vi "angle_sensor.vi"() -> (0 "Angle of system":dbl)   [LabVIEW 2014]
uses:
  <vilib>/myRIO/Instrument Drivers/Onboard IO/AI/typedefs/AI Reference.ctl
  <vilib>/myRIO/Common/Instrument Driver Framework/Utilities/typedefs/myRIO Generic Hardware Reference.ctl
  <vilib>/myRIO/Common/Instrument Driver Framework/Utilities/typedefs/Hardware Version Enum.ctl
  <vilib>/myRIO/Common/Instrument Driver Framework/Utilities/typedefs/myRIO v1.0 Reference.ctl
  <vilib>/myRIO/Common/Instrument Driver Framework/Utilities/typedefs/Generic FPGA Reference.ctl
  <vilib>/myRIO/Common/Instrument Driver Framework/myRIO v1.0/AI/typedefs/AI Channels List.ctl
  <vilib>/myRIO/Common/Instrument Driver Framework/myRIO v1.0/AI/typedefs/AI Channels Enum.ctl
  <vilib>/myRIO/Common/Instrument Driver Framework/Utilities/typedefs/Analog Scaling Constants List.ctl
  <vilib>/myRIO/Common/Instrument Driver Framework/Utilities/typedefs/Analog Scaling Constants.ctl
  <vilib>/userdefined/High Color/nirio_resource_hc.ctl
  <vilib>/myRIO/Common/Instrument Driver Framework/Utilities/vis/Is FPGA Ref Available.vi
  <vilib>/myRIO/Common/Instrument Driver Framework/myRIO v1.0/AI/vis/myRIO v1.1 Open AI.vi
  <vilib>/myRIO/Instrument Drivers/Onboard IO/AI/vis/Read.vi
  <vilib>/myRIO/Common/Instrument Driver Framework/Utilities/vis/Validate Channels.vi
  <vilib>/myRIO/Common/Instrument Driver Framework/myRIO v1.0/AI/vis/myRIO v1.0 Reserve AI.vi
  <vilib>/myRIO/Common/Instrument Driver Framework/myRIO v1.0/AI/vis/myRIO v1.0 Build MUX Configuration AI.vi
  <vilib>/myRIO/Common/Instrument Driver Framework/myRIO v1.0/Resource Manager/vis/myRIO v1.0 Reserve Channel List.vi
  <vilib>/myRIO/Common/Instrument Driver Framework/myRIO v1.0/Resource Manager/vis/myRIO v1.0 Reserve Channel.vi
  <vilib>/myRIO/Common/Instrument Driver Framework/myRIO v1.0/Resource Manager/vis/myRIO v1.0 Unreserve Channel.vi
  <vilib>/myRIO/Common/Instrument Driver Framework/myRIO v1.0/Resource Manager/vis/myRIO v1.0 Build Mutex Name.vi
  <vilib>/Utility/VariantDataType/GetNumericInfo.vi
  <vilib>/Utility/error.llb/Error Cluster From Error Code.vi
  <vilib>/myRIO/Common/Instrument Driver Framework/myRIO v1.0/myRIO v1.1 Open.vi
  <vilib>/myRIO/Common/Instrument Driver Framework/myRIO v1.0/AI/vis/myRIO v1.0 Get Scaling Constants AI.vi
  <vilib>/myRIO/Common/Instrument Driver Framework/Utilities/vis/IO Manager.vi
  <vilib>/myRIO/Common/Instrument Driver Framework/Utilities/vis/Configuration Manager.vi
  <vilib>/myRIO/Common/Instrument Driver Framework/myRIO v1.0/myRIO v1.0 Close.vi
  <vilib>/myRIO/Common/Instrument Driver Framework/myRIO v1.0/AI/vis/myRIO v1.0 Read AI.vi
  <vilib>/myRIO/Express VI/Onboard IO/AI/AI Express VI.xnode
  <vilib>/myRIO/Instrument Drivers/Onboard IO/AI/vis/myRIO AI Open.xnode
  <vilib>/myRIO/Instrument Drivers/Onboard IO/AI/AI.lvlib
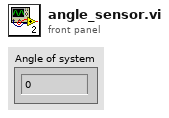
[diagram p1: front panel]
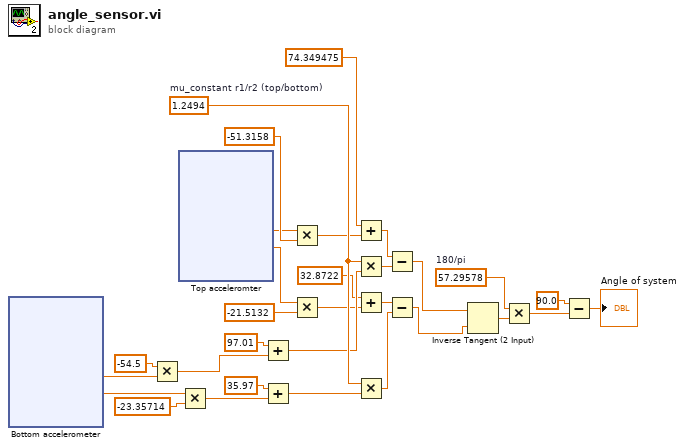
[diagram p0: block diagram]
diagram:
  w27 = 57.29578  # 180/pi
  w20 = 1.2494  # mu_constant r1/r2 (top/bottom)
  n1 = xnode "Bottom accelerometer"() -> ("x (C/AI0 (AI0))"=w9:dbl, "y (B/AI3 (Pin 9))"=w13:dbl)  [unwired: 1 in, 2 out]
  n2 = Multiply(x=-54.5, y=w9) -> (x*y=w11:dbl)
  n3 = xnode "Top acceleromter"() -> ("x (B/AI0 (Pin 3))"=w1:dbl, "y (B/AI1 (Pin 5))"=w5:dbl)  [unwired: 1 in, 2 out]
  n4 = Multiply(x=w13, y=-23.35714) -> (x*y=w15:dbl)
  n5 = Add(x=97.01, y=w11) -> (x+y=w17:dbl)
  n6 = Add(x=35.97, y=w15) -> (x+y=w21:dbl)
  n7 = Multiply(x=w1, y=-51.3158) -> (x*y=w3:dbl)
  n8 = Multiply(x=w5, y=-21.5132) -> (x*y=w7:dbl)
  n9 = Add(x=74.349475, y=w3) -> (x+y=w19:dbl)
  n10 = Multiply(x=w20, y=w17) -> (x*y=w18:dbl)
  n11 = Add(x=32.8722, y=w7) -> (x+y=w23:dbl)
  n12 = Multiply(x=w20, y=w21) -> (x*y=w22:dbl)
  n13 = Subtract(x=w19, y=w18) -> (x-y=w24:dbl)
  n14 = Subtract(x=w23, y=w22) -> (x-y=w25:dbl)
  n15 = Inverse Tangent (2 Input)(1:w25, 2:w24) -> (0:w26:dbl)
  n16 = Multiply(x=w27, y=w26) -> (x*y=w29:dbl)
  n17 = Subtract(x=90.0, y=w29) -> (x-y=→"Angle of system":dbl)
